vi "Running Average Using Stacked Shift Register.vi"() -> ()   [LabVIEW 2019]
uses:
  <vilib>/DAQmx/read.llb/DAQmx Read (Analog DBL 1Chan 1Samp).vi
  <vilib>/DAQmx/create/channels.llb/DAQmx Create Channel (AI-Temperature-Thermocouple).vi
  <vilib>/DAQmx/configure/timing.llb/DAQmx Timing (Sample Clock).vi
  <vilib>/DAQmx/miscellaneous.llb/DAQmx Fill In Error Info.vi
panel:
  in  "Stop":bool
  out "Average Temperature Chart":dbl(graph)
  out "Temperature Chart":dbl(graph)
  in  "Thermocouple Channel":tag="PCI-6221/ai0"
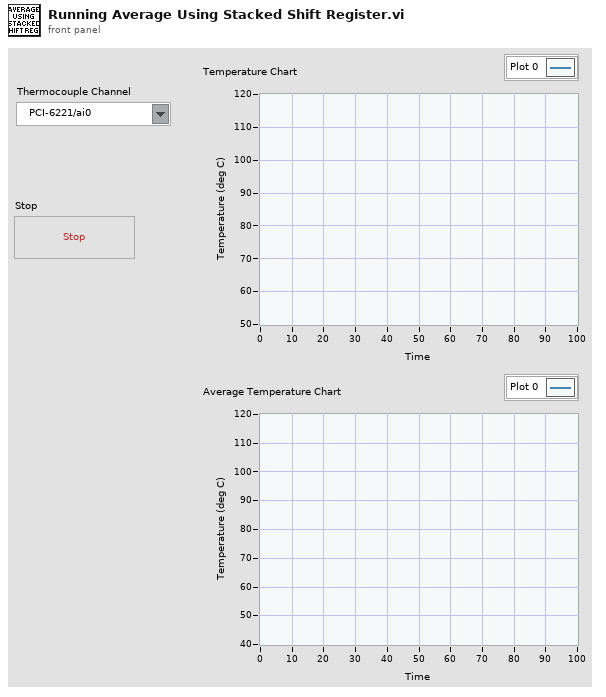
[diagram p1: front panel]
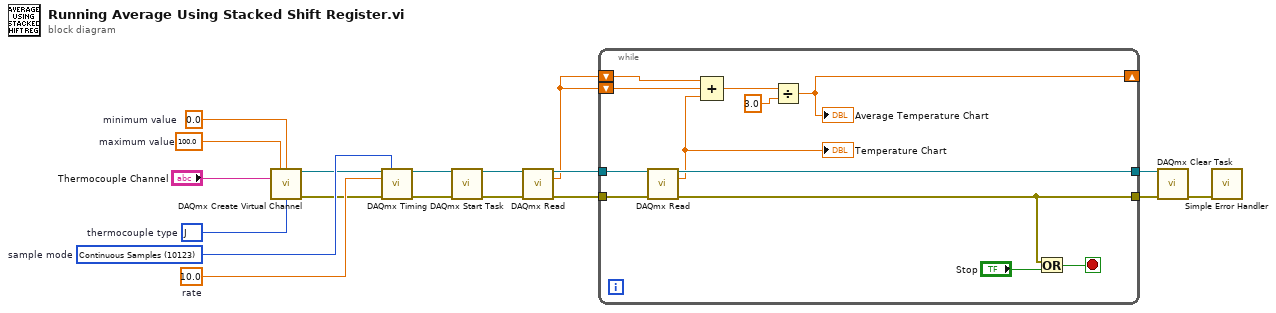
[diagram p0: block diagram]
diagram:
  w7 = 10072 items=["J"=10072, "K"=10073, "N"=10077, "R"=10082, "S"=10085, "T"=10086, "B"=10047, "E"=10055]  # thermocouple type
  w8 = 100.0  # maximum value
  w9 = 0.0  # minimum value
  w17 = 10.0  # rate
  w18 = 10123 items=["Finite Samples"=10178, "Continuous Samples"=10123, "Hardware Timed Single Point"=12522]  # sample mode
  n1 = call-poly <vilib>:"DAQmx Create Virtual Channel.vi"("maximum value"=w8, "minimum value"=w9, "physical channels"="Thermocouple Channel", "thermocouple type"=w7) -> ("task out"=w16:refnum<k21>, "error out"=w15:errorcluster)  [unwired: 10 in]
  n2 = call-poly <vilib>:"DAQmx Timing.vi"("task/channels in"=w16, "sample mode"=w18, "rate"=w17, "error in"=w15) -> ("task out"=w14:refnum<k21>, "error out"=w13:errorcluster)  [unwired: 10 in]
  n3 = call <vilib>:"DAQmx Start Task.vi"("task/channels in"=w14, "error in"=w13) -> ("task out"=w12:refnum<k21>, "error out"=w11:errorcluster)  [unwired: 12 in]
  n4 = call-poly <vilib>:"DAQmx Read.vi"("task/channels in"=w12, "error in"=w11) -> ("task out"=w6:refnum<k21>, "data"=w4:dbl, "error out"=w5:errorcluster)  [unwired: 11 in]
  n5 = while {
    tunnel: w6 -> [w30]
    tunnel: w5 -> [w29]
    shift-right: [w22] -> _
    shift-left: w4 -> [w28]
    shift-left: w4 -> [w27]
    tunnel: [w26] -> w3
    tunnel: [w21] -> w2
    stop <- w19 stop-if-true
    n6 = call-poly <vilib>:"DAQmx Read.vi"("task/channels in"=w30, "error in"=w29) -> ("task out"=w26:refnum<k21>, "data"=w23:dbl, "error out"=w21:errorcluster)  [unwired: 11 in]
    "Temperature Chart" <- w23
    n7 = Compound Arithmetic op=ADD(w28, w27, w23) -> (w25:dbl)
    n8 = Divide(x=w25, y=3.0) -> (x/y=w22:dbl)
    "Average Temperature Chart" <- w22
    n9 = Or(x=w21, y="Stop") -> (x .or. y?=w19:bool)
  }
  n10 = call <vilib>:"DAQmx Clear Task.vi"("task in"=w3, "error in"=w2) -> ("error out"=w1:errorcluster)  [unwired: 13 in]
  n11 = call <vilib>:"Simple Error Handler.vi"("error in (no error)"=w1) -> ()  [unwired: 4 in, 5 out]
